vi "PH_PSDBWriter.update Data Status Service.vi"(2 "Service ID":i32, 3 "Data Status":T1 items=["no info", "no Data collection", "no problem", "Error getting the ID", "Error writing Data", "Error getting the subsystem", "Error getting the Shot ID", "Error getting the Shot Types", "Error getting the Experiments", "Error verifying wanted Shottype", "Error verifying wanted Experiment"], 5 "error in (no error)":errorcluster) -> (19 "error out":errorcluster)   [LabVIEW 2014, in "PH_PSDBWriter.lvlib"]
doc: "By this VI a status service can be updated. For this purpose,\n\n0: no info\n1: no Data collection\n2: no problem\n3: Error getting the Instance ID\n4: Error writing Data to data base\n5: Error concerning the subsystem\n\ncan be selected."
uses:
  PH_PSDBWriter.lvlib
  PH_PSDBWriter.Data Status.ctl
  CSlibraries-extern/DimLVEvent/LVDimInterface/LVDimInterface.lvlib
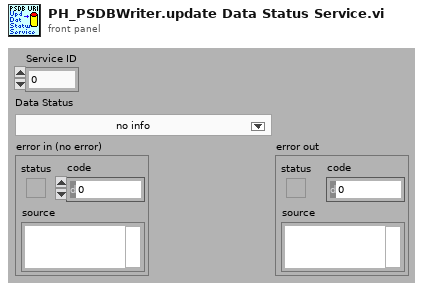
[diagram p1: front panel]
types:
  T1 = typedef "PH_PSDBWriter.lvlib/PH_PSDBWriter.Data Status.ctl" = i16
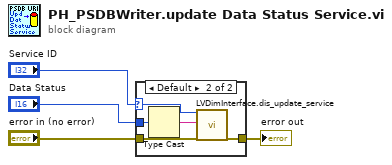
[diagram p0: block diagram]
diagram:
  n1 = case shown="Default" "Service ID" {
    selector: "Service ID" -> [_ w8]
    tunnel: [w5 w9] -> w4
    tunnel: "error in (no error)" -> [w5 w10]
    tunnel: "Data Status" -> [_ w6]
    frame -1 {
    }
    frame Default {
      n2 = Type Cast(x=w6) -> (*(type *) &x=w7:string)  [unwired: 1 in]
      n3 = call "LVDimInterface.dis_update_service.vi"("my_serviceID"=w8, "data"=w7, "error in (no error)"=w10) -> ("error out"=w9:errorcluster)  [unwired: 14 in, 2 out]
    }
  }
  "error out" <- w4
